vi "get zmq message stats.vi"(0 "message":string="{\"msg_id\":\"9\",\"msg_type\":\"read\",\"msg_property\":\"vset\",\"X\":X\"}", 11 "error in":errorcluster) -> (3 "Self Message":bool, 4 "msg_id":string, 6 "msg_type":string, 8 "msg_property":string, 10 "message dup":string="{\"msg_id\":\"9\",\"msg_type\":\"read\",\"msg_property\":\"vset\",\"X\":X\"}", 15 "error out":errorcluster)   [LabVIEW 2018]
uses:
  <vilib>/regexp/Match Regular Expression.xnode
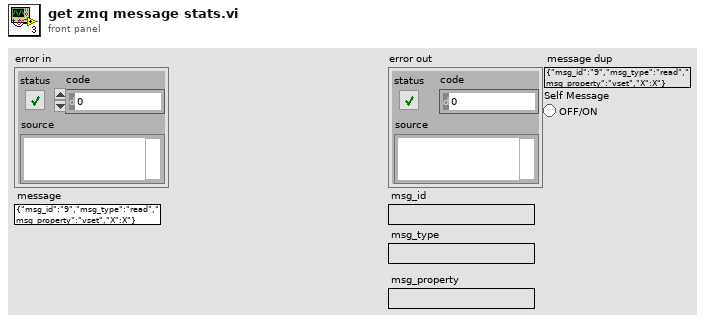
[diagram p1: front panel]
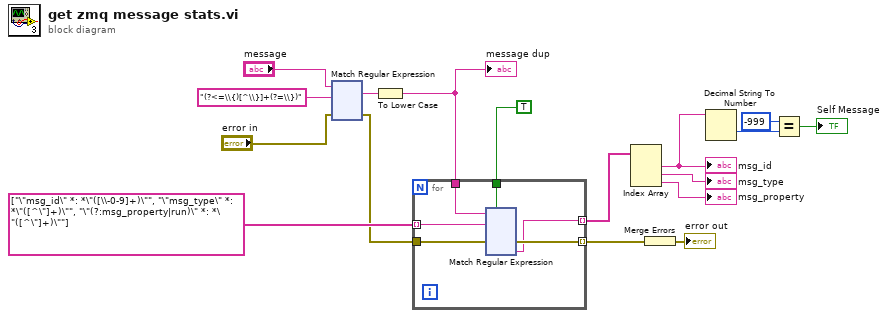
[diagram p0: block diagram]
diagram:
  n1 = xnode "Match Regular Expression"("input string"="message", "regular expression"="(?<=\\{)[^\\}]+(?=\\})", "error in"="error in") -> ("whole match"=w9:string, "error out"=w5:errorcluster)  [unwired: 3 in, 3 out]
  n2 = To Lower Case(string=w9) -> (all lower case string=w7:string)
  "message dup" <- w7
  n3 = for {
    tunnel: w7 -> [w23]
    tunnel: TRUE ("ignore case? (F)") -> [w22]
    tunnel: w5 -> [w21]
    tunnel: [w20] -> w16 mode=indexing
    tunnel: string[] ["\"msg_id\" *: *\"([\\-0-9]+)\"", "\"msg_type\" *: *\"([^\"]+)\"", "\"(?:msg_property|run)\" *: *\"([^\"]+)\""] -> [w19] mode=indexing
    tunnel: [w18] -> w13 mode=indexing
    n4 = xnode "Match Regular Expression"("input string"=w23, "regular expression"=w19, "error in"=w21, "ignore case? (F)"=w22) -> ("error out"=w20:errorcluster, "submatch 1"=w18:string)  [unwired: 2 in, 4 out]
  }
  n5 = Index Array(array=w13) -> (element #1=w4:string, element #2=→"msg_type":string, element #3=→"msg_property":string)  [unwired: 3 in]
  "msg_id" <- w4
  n6 = Merge Errors(w16) -> (→"error out":errorcluster)
  n7 = Decimal String To Number(string=w4) -> (number=w3:i32)  [unwired: 2 in, 1 out]
  n8 = Equal?(x=-999, y=w3) -> (x = y?=→"Self Message":bool)
